vi "Write Output Range.vi"(8 "error in (no error)":errorcluster, 10 "Output Range":T1, 11 "PID in":refnum<class "PID.lvclass">) -> (0 "error out":errorcluster, 3 "PID out":refnum<class "PID.lvclass">)   [LabVIEW 2020, in "IG PID.lvlib" / "PID.lvclass"]
uses:
  PID.lvclass
  Output Range.ctl
  PID.lvclass/PID.ctl
  IG PID.lvlib
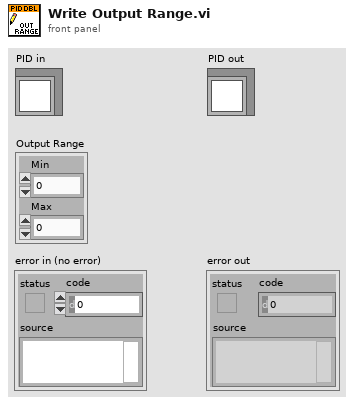
[diagram p1: front panel]
types:
  T1 = typedef "IG PID.lvlib/Output Range.ctl" = cluster{"Min":dbl, "Max":dbl}
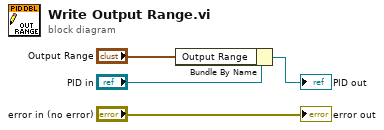
[diagram p0: block diagram]
diagram:
  n1 = Bundle By Name(cluster="PID in", "Output Range"="Output Range") -> (→"PID out":refnum<class "PID.lvclass">)
  "error out" <- "error in (no error)"
